vi "Spectrum_data_bundle_Jy_linear.vi"(6 "FFT size":dbl, 7 "Power spectrum input":dbl[](array[numeric]), 8 "dB_scale":bool caption="dB scale", 9 "Central frequency, Hz":dbl, 10 "Sample Rate":dbl, 11 "Plot mult":dbl) -> (3 "Output cluster to waveform graph":cluster{dbl, dbl, dbl[]})   [LabVIEW 2016]
doc: "The SubVI for preparing data for waveform graphs."
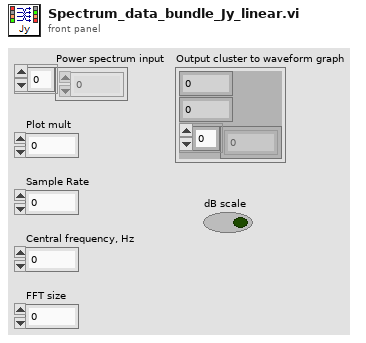
[diagram p1: front panel]
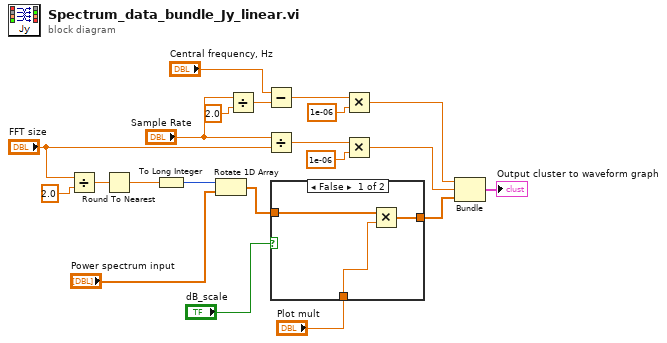
[diagram p0: block diagram]
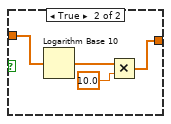
[diagram p2: hidden frame]
diagram:
  n1 = Divide(x="FFT size", y=2.0) -> (x/y=w4:dbl)
  n2 = Round To Nearest(number=w4) -> (nearest integer value=w5:dbl)
  n3 = To Long Integer(number=w5) -> (32bit integer=w14:i32)
  n4 = Rotate 1D Array(1:"Power spectrum input", 2:w14) -> (0:w3:dbl[])
  n5 = Divide(x="Sample Rate", y=2.0) -> (x/y=w12:dbl)
  n6 = Subtract(x="Central frequency, Hz", y=w12) -> (x-y=w13:dbl)
  n7 = Divide(x="Sample Rate", y="FFT size") -> (x/y=w10:dbl)
  n8 = case shown="False" "dB_scale" {
    tunnel: [w24 w25] -> w17
    tunnel: w3 -> [w23 w26]
    tunnel: "Plot mult" -> [w22 _]
    frame False {
      n9 = Multiply(x=w23, y=w22) -> (x*y=w24:dbl[])
    }
    frame True {
      n10 = Logarithm Base 10(1:w26) -> (0:w27:dbl[])
      n11 = Multiply(x=w27, y=10.0) -> (x*y=w25:dbl[])
    }
  }
  n12 = Multiply(x=w13, y=1e-06) -> (x*y=w16:dbl)
  n13 = Multiply(x=w10, y=1e-06 ("element")) -> (x*y=w8:dbl)
  n14 = Bundle(w16, w8, w17) -> (→"Output cluster to waveform graph":cluster{dbl, dbl, dbl[]})  [unwired: 1 in]
